vi "raptor_shutdown.vi"(8 "error in (no error)":errorcluster) -> (0 "error out":errorcluster)   [LabVIEW 2016]
doc: "Raptor: Shut down system."
uses:
  typedef/raptor_message.ctl
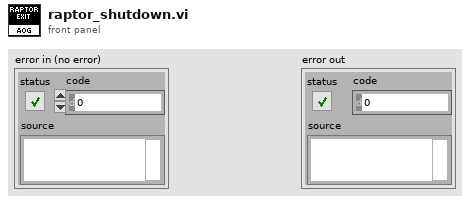
[diagram p1: front panel]
types:
  T1 = typedef "raptor_message.ctl" = cluster{"Message":enum16{"start", "stop", "initialise", "shutdown", "end scan", "new scan", "set depth"}, "Data":variant}
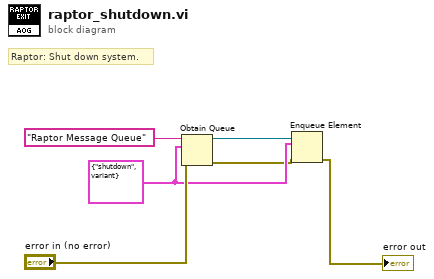
[diagram p0: block diagram]
diagram:
  w3 = T1 {"Message"=enum."shutdown", "Data"=variant} ("Cluster")
  # "Raptor: Shut down system."
  n1 = Obtain Queue(name (unnamed)="Raptor Message Queue", element data type=w3, error in (no error)="error in (no error)") -> (queue out=w4:refnum<queue>, error out=w2:errorcluster)  [unwired: 2 in, 1 out]
  n2 = Enqueue Element(queue=w4, element=w3, error in (no error)=w2) -> (error out=→"error out":errorcluster)  [unwired: 1 in, 2 out]
